vi "GLBL_STOP.vi"(10 "Stop":bool, 11 "Write_Read":bool) -> (2 "Stop out":bool)   [LabVIEW 2020]
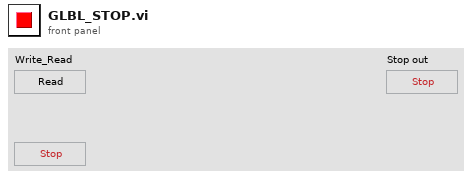
[diagram p1: front panel]
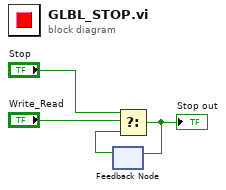
[diagram p0: block diagram]
diagram:
  n1 = feedback #1() -> (w2:bool)  [unwired: 1 in]
  n2 = Select(t="Stop", s="Write_Read", f=w2) -> (s? t:f=w1:bool)
  "Stop out" <- w1
  n3 = feedback-in #1(w1) -> ()
